vi "DB write for counter.vi"(2 "DB data":variant[][](array[variant]), 11 "DB write":T1) -> (6 "DB write":T2)   [LabVIEW 2015]
uses:
  <vilib>/addons/database/_DB Variant To Data/Database Variant To Data.xnode
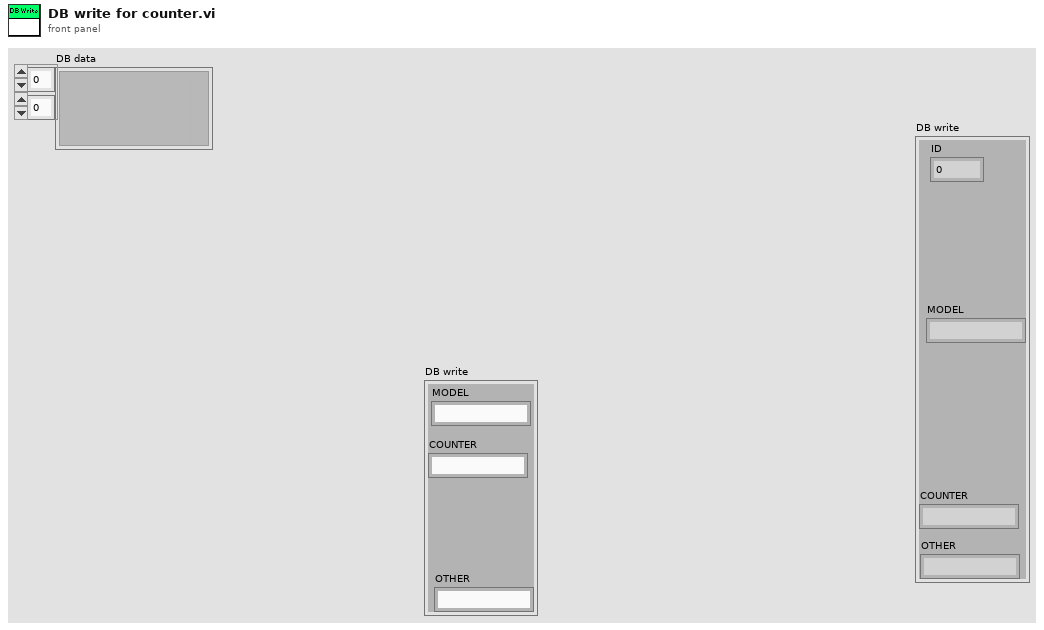
[diagram p1: front panel]
types:
  T1 = cluster{"MODEL":string, "COUNTER":string, "OTHER":string}
  T2 = cluster{"ID":i32, "MODEL":string, "COUNTER":string, "OTHER":string}
  T3 = cluster{i32, "MODEL":string, "COUNTER":string, "OTHER":string}
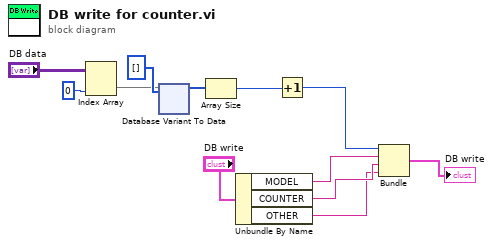
[diagram p0: block diagram]
diagram:
  n1 = Index Array(array="DB data", index (col)=0 ("disabled index (col)")) -> (element=w9:variant[])  [unwired: 1 in]
  n2 = xnode "Database Variant To Data"("database variant"=w9, "type"=i32[] []) -> ("data"=w10:i32[])  [unwired: 1 in, 1 out]
  n3 = Array Size(array=w10) -> (size(s)=w12:i32)
  n4 = Unbundle By Name("DB write") -> ("MODEL"=w4:string, "COUNTER"=w3:string, "OTHER"=w2:string)
  n5 = Increment(x=w12) -> (x+1=w6:i32)
  n6 = Bundle(w6, "MODEL"=w4, "COUNTER"=w3, "OTHER"=w2) -> (→"DB write":T3)  [unwired: 1 in]
